vi "30 Case Structure.vi"() -> ()   [LabVIEW 2018]
panel:
  in  "Add (F)/Subtract (T)":bool
  in  "stop":bool
  out "C":dbl
  in  "B":dbl
  in  "A":dbl
  # "Subtract"
  # "Add"
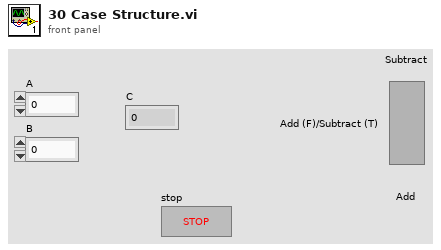
[diagram p1: front panel]
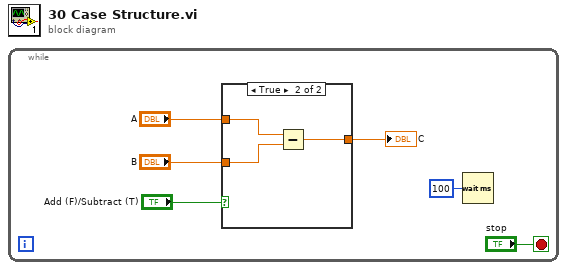
[diagram p0: block diagram]
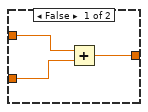
[diagram p2: hidden frame]
diagram:
  n1 = while {
    stop <- "stop" stop-if-true
    n2 = case shown="True" "Add (F)/Subtract (T)" {
      tunnel: "A" -> [w9 w12]
      tunnel: "B" -> [w8 w11]
      tunnel: [w7 w10] -> w4
      frame False {
        n3 = Add(x=w9, y=w8) -> (x+y=w7:dbl)
      }
      frame True {
        n4 = Subtract(x=w12, y=w11) -> (x-y=w10:dbl)
      }
    }
    "C" <- w4
    n5 = Wait (ms)(milliseconds to wait=u32 100) -> ()  [unwired: 1 out]
  }
